vi "InitResult.vi"(8 "error in (no error)":errorcluster, 10 "PGresult":u32, 11 "LibPath":path) -> (0 "error out":errorcluster, 3 "PQ Result out":refnum<class "PQ Result.lvclass">)   [LabVIEW 2016, in "PQ Result.lvclass"]
uses:
  PQ Result.lvclass
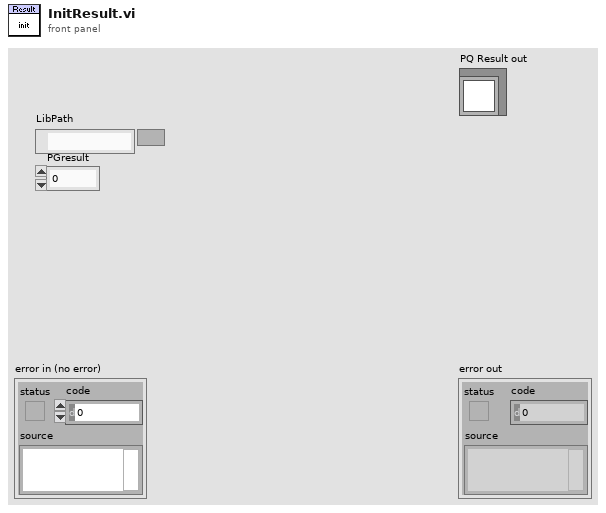
[diagram p1: front panel]
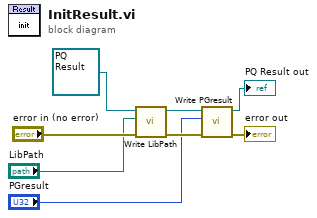
[diagram p0: block diagram]
diagram:
  n1 = call "Write LibPath.vi"("error in (no error)"="error in (no error)", "LibPath"="LibPath", "PQ Result in"=refnum<class "PQ Result.lvclass"> refnum ("PQ Result  in")) -> ("error out"=w3:errorcluster, "PQ Result out"=w4:refnum<class "PQ Result.lvclass">)  [unwired: 7 in]
  n2 = call "Write PGresult.vi"("error in (no error)"=w3, "PGresult"="PGresult", "PQ Result  in"=w4) -> ("error out"=→"error out":errorcluster, "PQ Result  out"=→"PQ Result out":refnum<class "PQ Result.lvclass">)  [unwired: 7 in]
